vi "RT Main.vi"   [LabVIEW 2018]
doc: "This template is for the Queued Message Handler design pattern.\n\nThe Event Handling Loop generates messages based on user interface actions.\n\nThe Message Handling Loop processes messages generated by the Event Handling Loop, or by other messages. The messages are string values, so new messages can be added easily to the Message Cases case structure in the Message Handling Loop. Each message cluster can also provide an optional value for Message Data, which is a variant that can be converted to whatever message-specific data is required."
uses:
  support/Message Queue/Message Queue.lvlib
  Globals/Global - All RT Loop Stop.vi
  <vilib>/rvi/interface/nirviReadWriteControl/nirviReadWriteControl.xnode
  controls/FPGA VI Reference.ctl
  <vilib>/rvi/errors/niLvFpgaAdjustHostInterfaceError.vi
  controls/FPGA State.ctl
  Globals/Global - Configuration Options.vi
  <vilib>/rvi/interface/nirviCloseFPGA/nirviCloseFPGA.xnode
  Globals/Global - RT Stream Connections.vi
  NiFpgaLv.dll
  <vilib>/rvi/interface/Simulation/niFpgaSimulationCallBeginRW.vi
  <vilib>/nisyscfg/nisyscfg.lvlib
  support/Message Queue/Message Cluster.ctl
  <vilib>/FPGAPlugInAG/Dynamic/niLvFpga_Close_Dynamic.vi
  controls/Sequence Engine State.ctl
  controls/Sequence Command.ctl
types:
  T1 = typedef "Sequence Command.ctl" = cluster{"Sequence Engine State":T2, "Message Data":variant}
  T2 = typedef "Sequence Engine State.ctl" = enum16{"Idle", "Running", "Stop", "Pause", "Resume", "Load Sequence"}
  T3 = typedef "FPGA VI Reference.ctl" = refnum<k20>
  T4 = typedef "FPGA State.ctl" = enum16{"Safe State", "Control (PID)"}
  T5 = typedef "Message Queue.lvlib/Message Cluster.ctl" = cluster{"Message":string, "Message Data":variant}
  T6 = cluster{"Sequence Engine State":T2, "Message Data":variant}
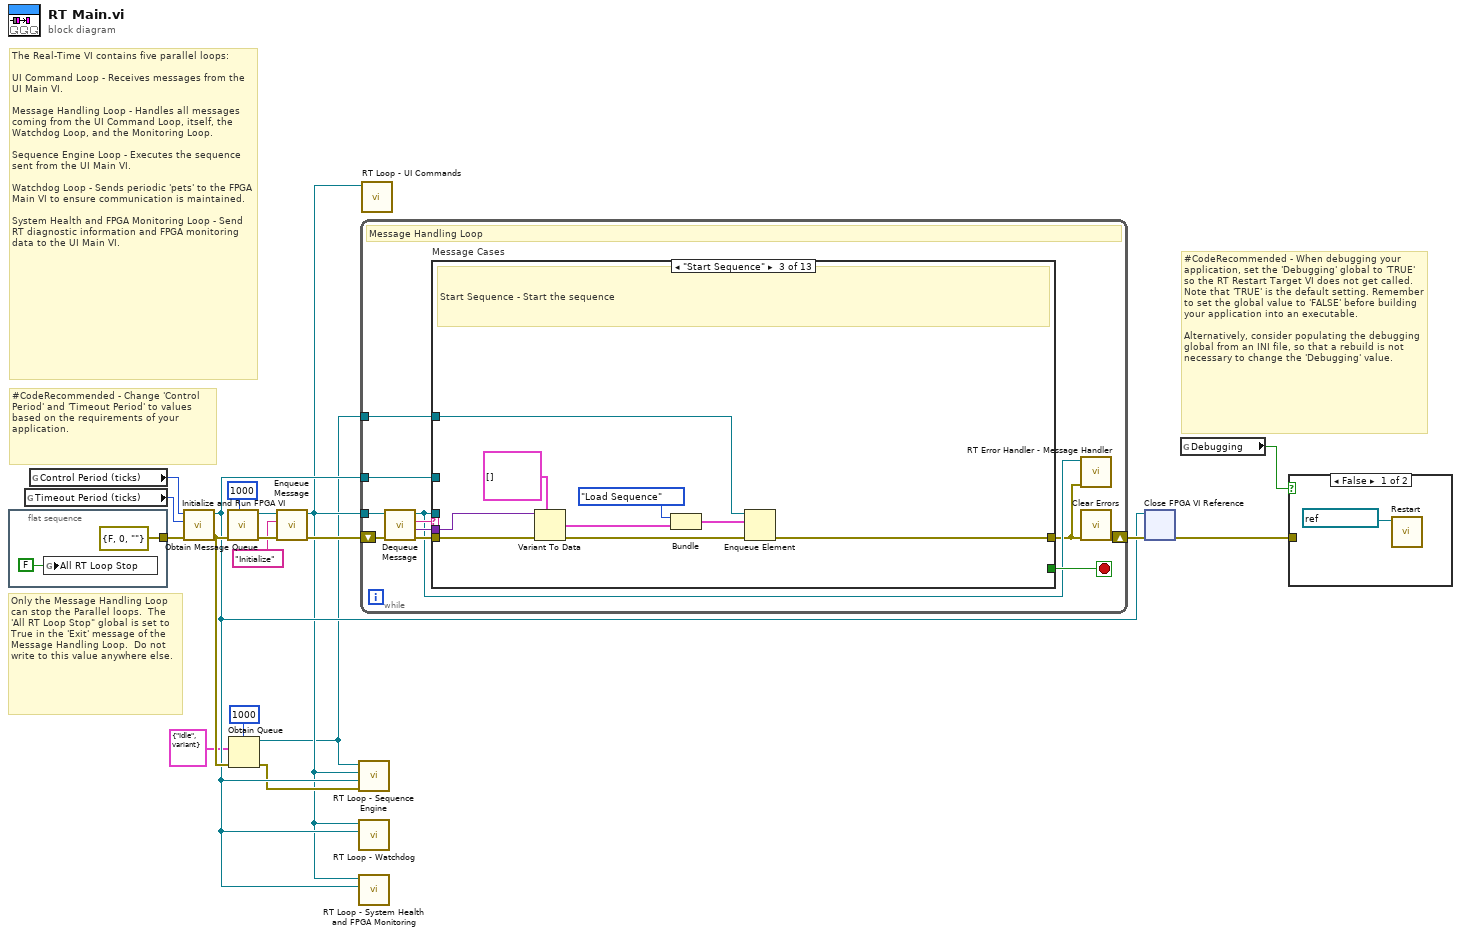
[diagram p0: block diagram]
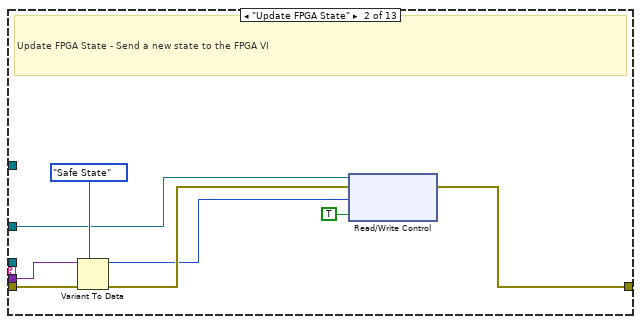
[diagram p4: hidden frame]
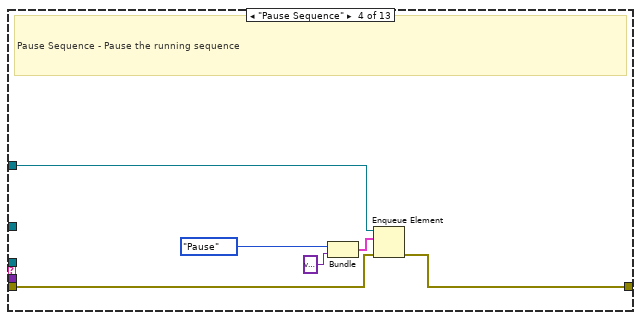
[diagram p5: hidden frame]
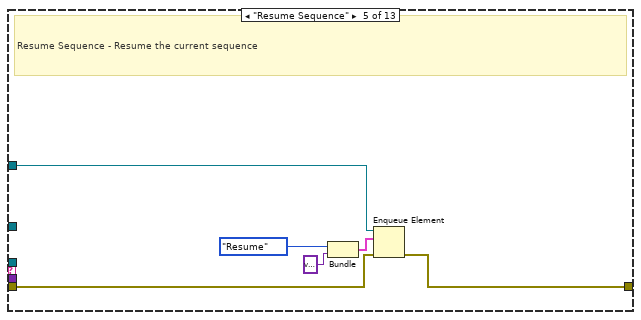
[diagram p6: hidden frame]
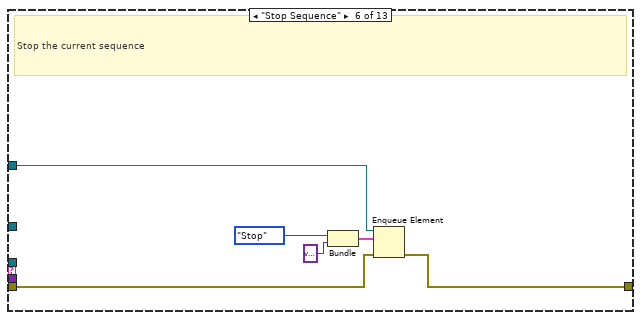
[diagram p7: hidden frame]
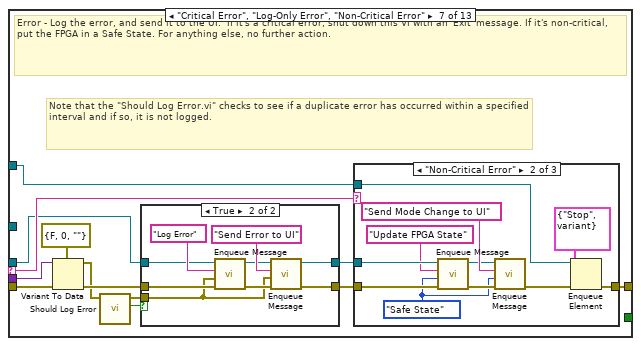
[diagram p8: hidden frame]
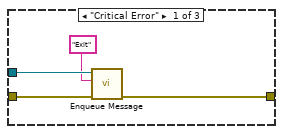
[diagram p10: hidden frame]
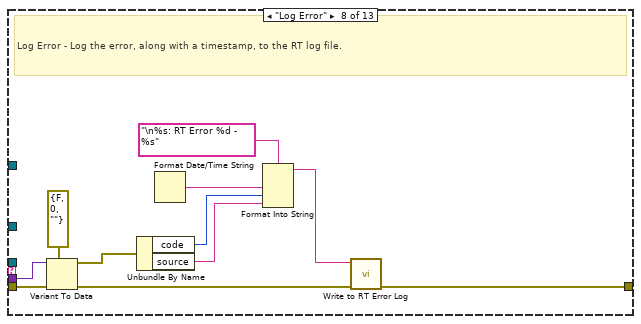
[diagram p12: hidden frame]
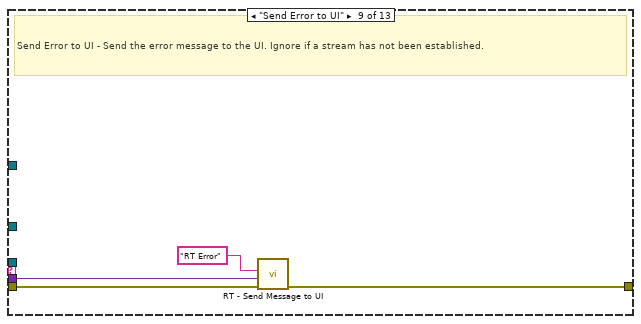
[diagram p13: hidden frame]
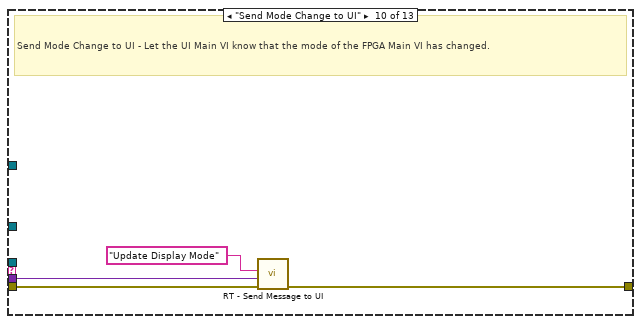
[diagram p14: hidden frame]
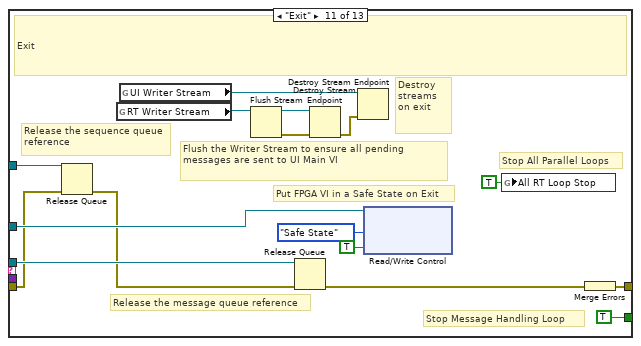
[diagram p15: hidden frame]
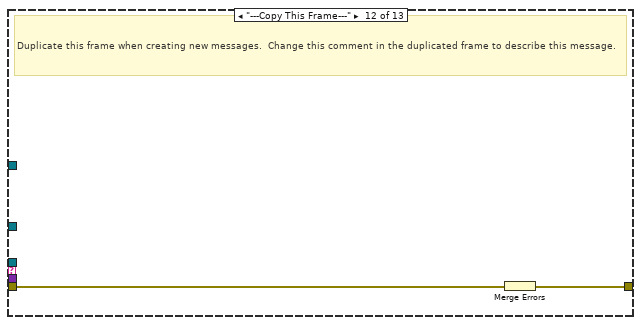
[diagram p16: hidden frame]
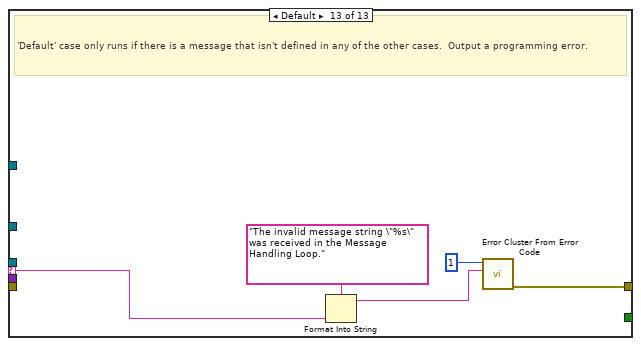
[diagram p17: hidden frame]
diagram:
  # "#CodeRecommended - When debugging your application, set the 'Debugging' global to 'TRUE' so the RT Restart Target VI does not get called.  Note that 'TRUE' is the default setting. Remember to set the global value to 'FALSE' before building your application into an executable.\n\nAlternatively, consider populating the debugging global from an INI file, so that a rebuild is not necessary to change the 'Debugging' value."
  # "#CodeRecommended - Change 'Control Period' and 'Timeout Period' to values based on the requirements of your application."
  # "The Real-Time VI contains five parallel loops:\n\nUI Command Loop - Receives messages from the UI Main VI.\n\nMessage Handling Loop - Handles all messages coming from the UI Command Loop, itself, the Watchdog Loop, and the Monitoring Loop.\n\nSequence Engine Loop - Executes the sequence sent from the UI Main VI.\n\nWatchdog Loop - Sends periodic 'pets' to the FPGA Main VI to ensure communication is maintained.\n\nSystem Health and FPGA Monitoring Loop - Send RT diagnostic information and FPGA monitoring data to the UI Main VI."
  # "Only the Message Handling Loop can stop the Parallel loops.  The 'All RT Loop Stop\" global is set to True in the 'Exit' message of the Message Handling Loop.  Do not write to this value anywhere else."
  n1 = flat-sequence {
    tunnel: [errorcluster {"status"=FALSE, "code"=0, "source"=""} ("error constant")] -> w14
    frame #0 {
      n2 = global write "Global - All RT Loop Stop.vi" "All RT Loop Stop"(FALSE) -> ()
    }
  }
  n3 = global read "Global - Configuration Options.vi" "Timeout Period (ticks)"() -> (w13:u64)
  n4 = global read "Global - Configuration Options.vi" "Control Period (ticks)"() -> (w12:u32)
  n5 = call "Initialize and Run FPGA VI.vi"("error in (no error)"=w14, "Timeout Period (ticks)"=w13, "Control Period (ticks)"=w12) -> ("error out"=w6:errorcluster, "FPGA VI Reference Out"=w5:T3)  [unwired: 7 in]
  n6 = call "Obtain Message Queue.vi"("max queue size (-1, unlimited)"=1000, "error in (no error)"=w6) -> ("error out"=w18:errorcluster, "Message Queue"=w17:refnum<queue>)  [unwired: 8 in]
  n7 = Obtain Queue(max queue size (-1, unlimited)=1000, element data type=T1 {"Sequence Engine State"=enum."Idle", "Message Data"=variant}, error in (no error)=w6) -> (queue out=w1:refnum<queue>, error out=w4:errorcluster)  [unwired: 2 in, 1 out]
  n8 = call "Enqueue Message.vi"("error in (no error)"=w18, "Message"="Initialize", "Message Queue"=w17) -> ("error out"=w15:errorcluster, "dup Message Queue"=w2:refnum<queue>)  [unwired: 7 in]
  n9 = call "RT Loop - Sequence Engine.vi"("error in (no error)"=w4, "FPGA VI Reference"=w5, "Message Queue"=w2, "Sequence Queue"=w1) -> ()  [unwired: 8 in]
  n10 = call "RT Loop - Watchdog.vi"("FPGA VI Reference"=w5, "Message Queue"=w2) -> ()  [unwired: 10 in]
  n11 = call "RT Loop - System Health and FPGA Monitoring.vi"("FPGA VI Reference"=w5, "Message Queue"=w2) -> ()  [unwired: 10 in]
  n12 = while {
    tunnel: w2 -> [w26]
    shift-right: [w23] -> w11
    shift-left: w15 -> [w30]
    tunnel: w5 -> [w25]
    tunnel: w1 -> [w21]
    stop <- w31 stop-if-true
    # "Message Handling Loop"
    n13 = call "Dequeue Message.vi"("error in (no error)"=w30, "Message Queue"=w26) -> ("error out"=w29:errorcluster, "Message Data"=w27:variant, "Message"=w28:string, "dup Message Queue"=w24:refnum<queue>)  [unwired: 6 in]
    n14 = case "Message Cases" shown="\"Start Sequence\"" w28 {
      selector: w28 -> [_ _ _ _ _ _ w78 _ _ _ _ _ w148]
      tunnel: w24 -> [_ _ _ _ _ _ w72 _ _ _ w142 _ _]
      tunnel: w29 -> [w32 w40 w44 w53 w59 w65 w76 w118 w122 w126 w128 w144 _]
      tunnel: [w32 w37 w42 w55 w61 w67 w77 w109 w119 w125 w139 w143 w146] -> w22
      tunnel: [_ _ _ _ _ _ _ _ _ _ TRUE _ _] -> w31
      tunnel: w27 -> [_ w39 w49 _ _ _ w75 w117 w121 w124 _ _ _]
      tunnel: w25 -> [_ w35 _ _ _ _ _ _ _ _ w135 _ _]
      tunnel: w21 -> [_ _ w41 w54 w60 w66 w68 _ _ _ w129 _ _]
      frame "Initialize" {
        # "Initialize - Currently a no-op for the RT Main VI"
      }
      frame "Update FPGA State" {
        # "Update FPGA State - Send a new state to the FPGA VI"
        n15 = Variant To Data(error in=w40, type=FPGA_State."Safe State" ("FPGA State"), Variant=w39) -> (data=w34:T4, error out=w36:errorcluster)
        n16 = xnode "Read/Write Control"("FPGA VI Reference In"=w35, "error in"=w36, "New State"=w34, "Change State"=TRUE) -> ("error out"=w37:errorcluster)  [unwired: 1 out]
      }
      frame "Start Sequence" {
        # "Start Sequence - Start the sequence"
        n17 = Variant To Data(error in=w44, type=T5[] [], Variant=w49) -> (data=w47:T5[], error out=w43:errorcluster)
        n18 = Bundle("Sequence Engine State"=Sequence_Engine_State."Load Sequence", w47) -> (w45:cluster{"Sequence Engine State":T2, T5[]})  [unwired: 1 in]
        n19 = Enqueue Element(queue=w41, element=w45, error in (no error)=w43) -> (error out=w42:errorcluster)  [unwired: 1 in, 2 out]
      }
      frame "Pause Sequence" {
        # "Pause Sequence - Pause the running sequence"
        n20 = Bundle("Sequence Engine State"=Sequence_Engine_State."Pause", "Message Data"=variant) -> (w50:T6)  [unwired: 1 in]
        n21 = Enqueue Element(queue=w54, element=w50, error in (no error)=w53) -> (error out=w55:errorcluster)  [unwired: 1 in, 2 out]
      }
      frame "Resume Sequence" {
        # "Resume Sequence - Resume the current sequence"
        n22 = Bundle("Sequence Engine State"=Sequence_Engine_State."Resume", "Message Data"=variant) -> (w56:T6)  [unwired: 1 in]
        n23 = Enqueue Element(queue=w60, element=w56, error in (no error)=w59) -> (error out=w61:errorcluster)  [unwired: 1 in, 2 out]
      }
      frame "Stop Sequence" {
        # "Stop the current sequence"
        n24 = Bundle("Sequence Engine State"=Sequence_Engine_State."Stop", "Message Data"=variant) -> (w62:T6)  [unwired: 1 in]
        n25 = Enqueue Element(queue=w66, element=w62, error in (no error)=w65) -> (error out=w67:errorcluster)  [unwired: 1 in, 2 out]
      }
      frame "Critical Error", "Log-Only Error", "Non-Critical Error" {
        # "Note that the \"Should Log Error.vi\" checks to see if a duplicate error has occurred within a specified interval and if so, it is not logged."
        # "Error - Log the error, and send it to the UI.  If it's a critical error, shut down this VI with an 'Exit' message. If it's non-critical, put the FPGA in a Safe State. For anything else, no further action."
        n26 = Variant To Data(error in=w76, type=errorcluster {"status"=FALSE, "code"=0, "source"=""} ("error out"), Variant=w75) -> (data=w70:errorcluster, error out=w73:errorcluster)
        n27 = call "Should Log Error.vi"("error to report"=w70) -> ("Should Log Error?"=w71:bool, "dup error to report"=w69:errorcluster)  [unwired: 9 in]
        n28 = case shown="True" w71 {
          tunnel: [w82 w89] -> w80
          tunnel: [w81 w88] -> w79
          tunnel: w72 -> [w81 w87]
          tunnel: w73 -> [w82 w84]
          tunnel: w69 -> [_ w83]
          frame False {
          }
          frame True {
            n29 = call "Enqueue Message.vi"("error in (no error)"=w84, "Message Data"=w83, "Message"="Log Error", "Message Queue"=w87) -> ("error out"=w85:errorcluster, "dup Message Queue"=w86:refnum<queue>)  [unwired: 6 in]
            n30 = call "Enqueue Message.vi"("error in (no error)"=w85, "Message Data"=w83, "Message"="Send Error to UI", "Message Queue"=w86) -> ("error out"=w89:errorcluster, "dup Message Queue"=w88:refnum<queue>)  [unwired: 6 in]
          }
        }
        n31 = case shown="\"Non-Critical Error\"" w78 {
          tunnel: w80 -> [w95 w106 w107]
          tunnel: w79 -> [w93 w105 _]
          tunnel: [w94 w98 w107] -> w77
          tunnel: w68 -> [_ w97 _]
          frame "Critical Error" {
            n32 = call "Enqueue Message.vi"("error in (no error)"=w95, "Message"="Exit", "Message Queue"=w93) -> ("error out"=w94:errorcluster)  [unwired: 7 in, 1 out]
          }
          frame "Non-Critical Error" {
            w100 = FPGA_State."Safe State" ("FPGA State")
            n33 = call "Enqueue Message.vi"("error in (no error)"=w106, "Message Data"=w100, "Message"="Update FPGA State", "Message Queue"=w105) -> ("error out"=w103:errorcluster, "dup Message Queue"=w101:refnum<queue>)  [unwired: 6 in]
            n34 = call "Enqueue Message.vi"("error in (no error)"=w103, "Message Data"=w100, "Message"="Send Mode Change to UI", "Message Queue"=w101) -> ("error out"=w99:errorcluster)  [unwired: 6 in, 1 out]
            n35 = Enqueue Element(queue=w97, element=T1 {"Sequence Engine State"=enum."Stop", "Message Data"=variant}, error in (no error)=w99) -> (error out=w98:errorcluster)  [unwired: 1 in, 2 out]
          }
          frame Default {
          }
        }
      }
      frame "Log Error" {
        # "Log Error - Log the error, along with a timestamp, to the RT log file."
        n36 = Variant To Data(error in=w118, type=errorcluster {"status"=FALSE, "code"=0, "source"=""} ("error constant"), Variant=w117) -> (data=w112:errorcluster, error out=w115:errorcluster)
        n37 = Unbundle By Name(w112) -> ("code"=w111:i32, "source"=w110:string)
        n38 = Format Date/Time String() -> (date/time string=w113:string)  [unwired: 3 in]
        n39 = Format Into String(format string="\n%s: RT Error %d - %s", w113, w111, w110) -> (resulting string=w108:string)  [unwired: 2 in, 1 out]
        n40 = call "Write to RT Error Log.vi"("error in (no error)"=w115, "Log Entry"=w108) -> ("error out"=w109:errorcluster)  [unwired: 9 in]
      }
      frame "Send Error to UI" {
        # "Send Error to UI - Send the error message to the UI. Ignore if a stream has not been established."
        n41 = call "RT - Send Message to UI.vi"("error in (no error)"=w122, "Message Data"=w121, "Message"="RT Error") -> ("error out"=w119:errorcluster)  [unwired: 8 in]
      }
      frame "Send Mode Change to UI" {
        # "Send Mode Change to UI - Let the UI Main VI know that the mode of the FPGA Main VI has changed."
        n42 = call "RT - Send Message to UI.vi"("error in (no error)"=w126, "Message Data"=w124, "Message"="Update Display Mode") -> ("error out"=w125:errorcluster)  [unwired: 8 in]
      }
      frame "Exit" {
        # "Release the sequence queue reference"
        # "Flush the Writer Stream to ensure all pending messages are sent to UI Main VI"
        # "Destroy streams on exit"
        # "Put FPGA VI in a Safe State on Exit"
        # "Stop Message Handling Loop"
        # "Stop All Parallel Loops"
        # "Release the message queue reference"
        # "Exit"
        n43 = Release Queue(queue=w129, error in (no error)=w128) -> (error out=w127:errorcluster)  [unwired: 1 in, 2 out]
        n44 = global read "Global - RT Stream Connections.vi" "RT Writer Stream"() -> (w132:refnum<k21>)
        n45 = global read "Global - RT Stream Connections.vi" "UI Writer Stream"() -> (w134:refnum<k21>)
        n46 = Flush Stream(11:w132) -> (0:w130:errorcluster, 3:w131:refnum<k21>)  [unwired: 3 in, 1 out]
        n47 = Release Queue(queue=w142, error in (no error)=w127) -> (error out=w140:errorcluster)  [unwired: 1 in, 2 out]
        n48 = Destroy Stream Endpoint(8:w130, 11:w131) -> (0:w133:errorcluster)
        n49 = Destroy Stream Endpoint(8:w133, 11:w134) -> ()  [unwired: 1 out]
        n50 = xnode "Read/Write Control"("FPGA VI Reference In"=w135, "New State"=FPGA_State."Safe State", "Change State"=TRUE) -> ()  [unwired: 1 in, 2 out]
        n51 = global write "Global - All RT Loop Stop.vi" "All RT Loop Stop"(TRUE ("Stop Monitoring Loops")) -> ()
        n52 = Merge Errors(w140) -> (w139:errorcluster)
      }
      frame "---Copy This Frame---" {
        # "Duplicate this frame when creating new messages.  Change this comment in the duplicated frame to describe this message."
        n53 = Merge Errors(w144) -> (w143:errorcluster)
      }
      frame Default {
        # "'Default' case only runs if there is a message that isn't defined in any of the other cases.  Output a programming error."
        n54 = Format Into String(format string="The invalid message string \"%s\" was received in the Message Handling Loop." ("Unknown Message Error Text"), w148) -> (resulting string=w145:string)  [unwired: 2 in, 1 out]
        n55 = call <vilib>:"Error Cluster From Error Code.vi"("error message (\"\")"=w145, "error code (0)"=1) -> ("error out"=w146:errorcluster)  [unwired: 7 in]
      }
    }
    n56 = call "RT Error Handler - Message Handler.vi"("error in (no error)"=w22, "Message Queue"=w24) -> ()  [unwired: 9 in, 1 out]
    n57 = call <vilib>:"Clear Errors.vi"("error in (no error)"=w22) -> ("error out"=w23:errorcluster)  [unwired: 5 in, 1 out]
  }
  n58 = call "RT Loop - UI Commands.vi"("Message Queue"=w2) -> ()  [unwired: 11 in]
  n59 = xnode "Close FPGA VI Reference"("FPGA VI Reference In"=w5, "error in"=w11) -> ("error out"=w10:errorcluster)
  n60 = global read "Global - Configuration Options.vi" "Debugging"() -> (w9:bool)
  n61 = case shown="False" w9 {
    tunnel: w10 -> [_ _]
    frame False {
      n62 = call <vilib>:"Restart.vi"("Session in"=refnum<k21> "localhost" ("session in")) -> ()  [unwired: 8 in, 3 out]
    }
    frame True {
    }
  }
